vi "Process FCT Request.vi"(11 "FHPP in":refnum<class "FHPP.lvclass">) -> (3 "FHPP out":refnum<class "FHPP.lvclass">)   [LabVIEW 2022 SP3, in "FHPP.lvclass"]
uses:
  FHPP.lvclass
  FHPP.lvclass/FHPP.ctl
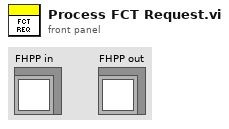
[diagram p1: front panel]
types:
  T1 = typedef "FHPP.lvclass/FCT Request.ctl" = cluster{"Request":T2, "PNU":u16, "Subindex":u16, "Data":u32}
  T2 = typedef "FHPP.lvclass/ReqID.ctl" = u8
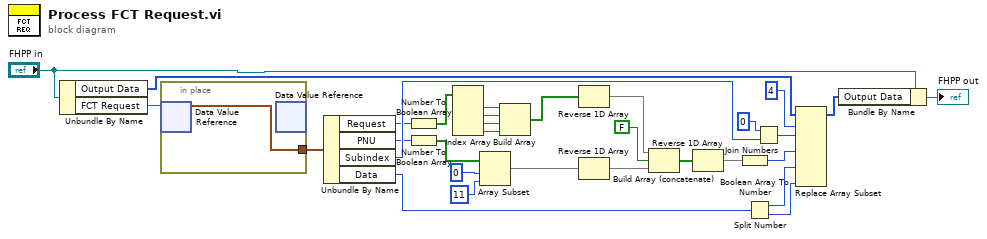
[diagram p0: block diagram]
diagram:
  n1 = Unbundle By Name("FHPP in") -> ("Output Data"=w29:u16[], "FCT Request"=w30:refnum<data-value>)
  n2 = in-place {
    in-place-border: [w32] -> w31
    n3 = in-place-dvr #1(w30) -> (w32:T1)  [unwired: 1 out]
    n4 = in-place-dvr #1() -> ()  [unwired: 1 in, 2 out]
  }
  n5 = Unbundle By Name(w31) -> ("Request"=w20:T2, "PNU"=w21:u16, "Subindex"=w22:u16, "Data"=w23:u32)
  n6 = Number To Boolean Array(number=w20) -> (Boolean array=w7:bool[])
  n7 = Number To Boolean Array(number=w21) -> (Boolean array=w2:bool[])
  n8 = Index Array(array=w7) -> (element #1=w8:bool, element #2=w9:bool, element #3=w10:bool, element #4=w11:bool)  [unwired: 4 in]
  n9 = Array Subset(array=w2, index=0, length=11) -> (w13:bool[])
  n10 = Build Array(w8, w9, w10, w11) -> (w12:bool[])
  n11 = Reverse 1D Array(array=w12) -> (reversed array=w15:bool[])
  n12 = Reverse 1D Array(array=w13) -> (reversed array=w16:bool[])
  n13 = Build Array (concatenate)(w15, FALSE ("element"), w16) -> (w5:bool[])
  n14 = Reverse 1D Array(array=w5) -> (reversed array=w14:bool[])
  n15 = Boolean Array To Number(Boolean array=w14) -> (number=w6:u16)
  n16 = Split Number(x=w23) -> (hi(x)=w24:u16, lo(x)=w25:u16)
  n17 = Join Numbers(hi=u16 0, lo=w22) -> ((hi.lo)=w18:u32)
  n18 = Replace Array Subset(array=w29, new element #1=w18, index #1=4 ("index"), new element #2=w6, new element #3=w24, new element #4=w25) -> (w27:u16[])  [unwired: 3 in]
  n19 = Bundle By Name(cluster="FHPP in", "Output Data"=w27) -> (→"FHPP out":refnum<class "FHPP.lvclass">)
